vi "Search Array.vi"(3 "abbrev":string, 4 "instrarray":T1(array[cluster])) -> (0 "index":i32, 1 "on?":bool, 2 "found?":bool)   [LabVIEW 2009, in "Magnet.lvclass"]
uses:
  Magnet.lvclass
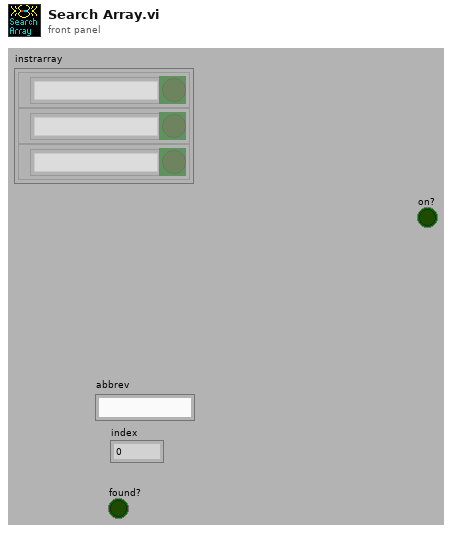
[diagram p1: front panel]
types:
  T1 = cluster{"name":string, "on?":bool, "abbrev":string}[]
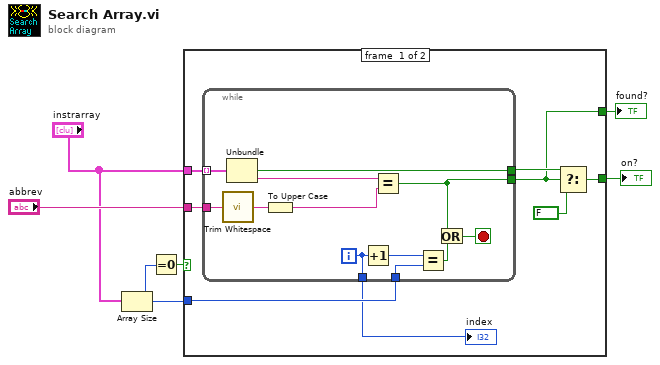
[diagram p0: block diagram]
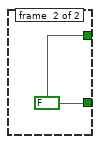
[diagram p2: hidden frame]
diagram:
  n1 = Array Size(array="instrarray") -> (size(s)=w2:i32)
  n2 = Equal To 0?(x=w2) -> (x = 0?=w3:bool)
  n3 = case shown="False" w3 {
    tunnel: "abbrev" -> [w14 _]
    tunnel: w2 -> [w13 _]
    tunnel: [w10 w27] -> w5
    tunnel: "instrarray" -> [w9 _]
    tunnel: [w7 w27] -> w1
    frame #0 {
      n4 = while {
        tunnel: w9 -> [w25] mode=indexing
        tunnel: w14 -> [w26]
        tunnel: [w22] -> w12
        tunnel: w13 -> [w21]
        tunnel: [w18] -> w7
        tunnel: [w15] -> w8
        i -> [w15]
        stop <- w19 stop-if-true
        n5 = call <vilib>:"Trim Whitespace.vi"("string"=w26) -> ("trimmed string"=w24:string)  [unwired: 1 in]
        n6 = Unbundle(w25) -> ("on?"=w22:bool, "abbrev"=w23:string)  [unwired: 1 out]
        n7 = To Upper Case(1:w24) -> (0:w16:string)
        n8 = Increment(x=w15) -> (x+1=w17:i32)
        n9 = Equal?(x=w23, y=w16) -> (x = y?=w18:bool)
        n10 = Equal?(x=w17, y=w21) -> (x = y?=w20:bool)
        n11 = Or(x=w18, y=w20) -> (x .or. y?=w19:bool)
      }
      "index" <- w8
      n12 = Select(t=w12, s=w7, f=FALSE) -> (s? t:f=w10:bool)
    }
    frame #1 {
      w27 = FALSE
    }
  }
  "on?" <- w5
  "found?" <- w1
